vi "ServoConditioning.vi"(11 "servo input":i16) -> (3 "output":u16)   [LabVIEW 2010, in "kevLib2011.lvlib"]
uses:
  kevLib2011.lvlib
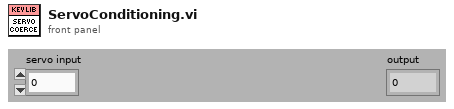
[diagram p1: front panel]
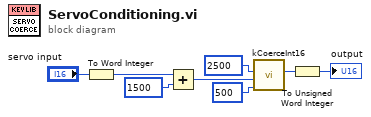
[diagram p0: block diagram]
diagram:
  n1 = To Word Integer(number="servo input") -> (16bit integer=w3:i16)
  n2 = Add(x=w3, y=i16 1500) -> (x+y=w7:i16)
  n3 = call "kCoerceInt16.vi"("lower"=i16 500, "input"=w7, "upper"=i16 2500) -> ("output"=w2:i16)  [unwired: 7 in, 1 out]
  n4 = To Unsigned Word Integer(number=w2) -> (unsigned 16bit integer=→"output":u16)
